vi "propactivex.vi"   [LabVIEW 2014]
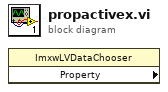
[diagram p0: block diagram]
diagram:
  n1 = property class="ImxwLVDataChooser" props=[]() -> ()  [unwired: 2 in, 3 out]
